vi "Kill BFECC.vi"(8 "error in (no error)":errorcluster, 11 "BFECC in":refnum<class "BFECC.lvclass">) -> (0 "error out":errorcluster, 3 "BFECC out":refnum<class "BFECC.lvclass">)   [LabVIEW 2018, in "BFECC.lvlib" / "BFECC.lvclass"]
doc: "Close all BFECC Windows that have been opened."
uses:
  BFECC.lvclass
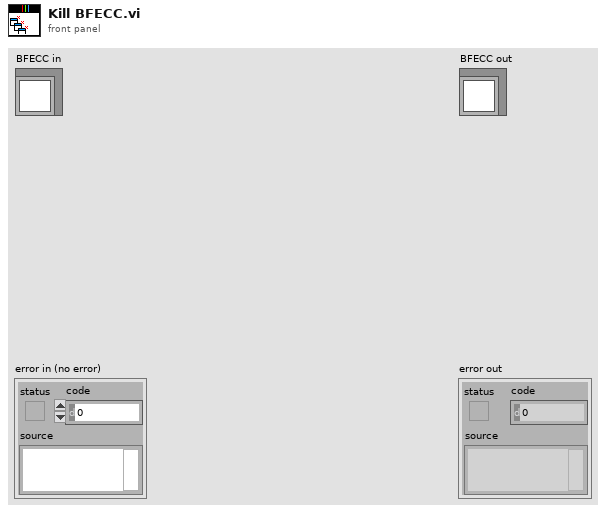
[diagram p1: front panel]
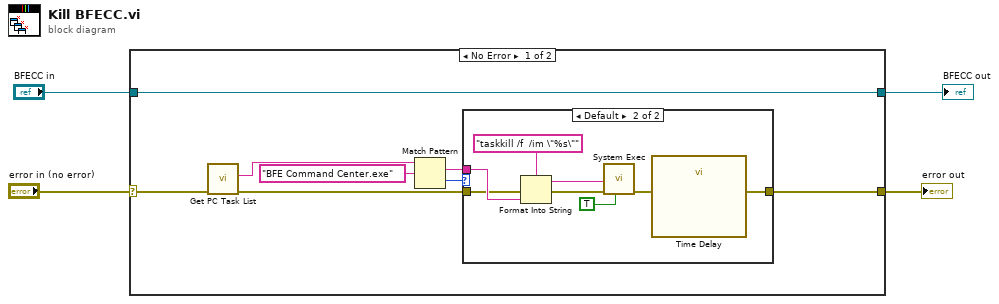
[diagram p0: block diagram]
diagram:
  n1 = case shown="No Error" "error in (no error)" {
    selector: "error in (no error)" -> [w12 w23]
    tunnel: [w6 w23] -> w3
    tunnel: [w7 w22] -> w1
    tunnel: "BFECC in" -> [w7 w22]
    frame No Error {
      n2 = call "Get PC Task List.vi"("error in (no error)"=w12) -> ("error out"=w8:errorcluster, "Tasklist"=w11:string)  [unwired: 9 in]
      n3 = Match Pattern(string=w11, regular expression="BFE Command Center.exe") -> (match substring=w9:string, offset past match=w5:i32)  [unwired: 1 in, 2 out]
      n4 = case shown="Default" w5 {
        tunnel: w9 -> [_ w21]
        tunnel: w8 -> [w13 w19]
        tunnel: [w13 w14] -> w6
        frame -1 {
        }
        frame Default {
          n5 = Format Into String(format string="taskkill /f  /im \"%s\"", error in=w19, w21) -> (resulting string=w17:string, error out=w18:errorcluster)  [unwired: 1 in]
          n6 = call <vilib>:"System Exec.vi"("run minimized? (F)"=TRUE, "error in (no error)"=w18, "command line"=w17) -> ("error out"=w15:errorcluster)  [unwired: 5 in, 3 out]
          n7 = call "Time Delay"("error in (no error)"=w15) -> ("error out"=w14:errorcluster)  [unwired: 10 in]
        }
      }
    }
    frame Error {
    }
  }
  "error out" <- w3
  "BFECC out" <- w1
